vi "Handle ePhys.vi"(9 "Amplification Factor":dbl, 10 "Use Ephys":bool, 11 "data":dbl[][](array[numeric])) -> ()   [LabVIEW 2018]
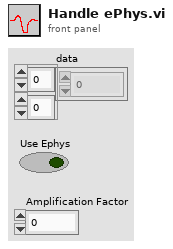
[diagram p1: front panel]
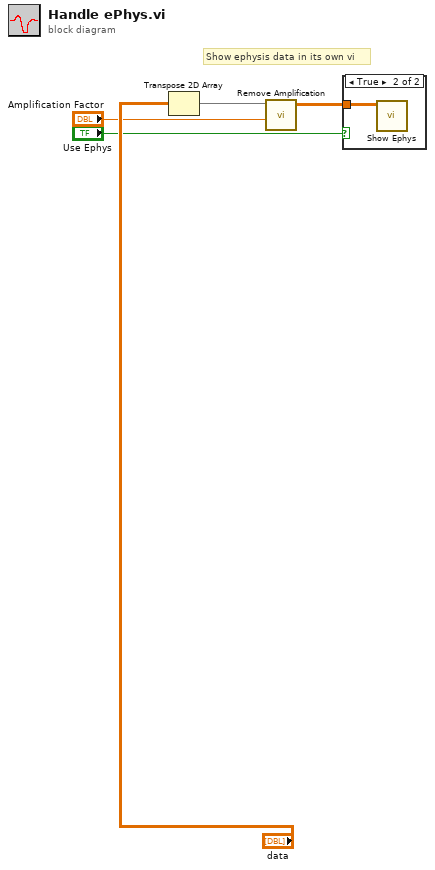
[diagram p0: block diagram]
diagram:
  # "Show ephysis data in its own vi"
  n1 = Transpose 2D Array(2D array="data") -> (transposed array=w4:dbl[][])
  n2 = call "Remove Amplification.vi"("Amplification Factor"="Amplification Factor", "Array"=w4) -> ("Array 2"=w2:dbl[][])  [unwired: 9 in]
  n3 = case shown="True" "Use Ephys" {
    tunnel: w2 -> [_ w6]
    frame False {
    }
    frame True {
      n4 = call "Show Ephys.vi"("Array"=w6) -> ()  [unwired: 11 in]
    }
  }
